vi "Create FTP Connection.vi"(8 "error in (no error)":errorcluster caption="错误输入（无错误）") -> (0 "error out":errorcluster caption="错误输出", 3 "TCP网络连接输出":T1)   [LabVIEW 2013]
uses:
  <vilib>/FTP/ftp0.llb/FTP Session.ctl
  <vilib>/FTP/NI_FTP.lvlib
panel:
  in  "port (21)":u16=21 caption="端口(21)"
  in  "password":string="success" caption="密码"
  in  "user":string="SUN Shouwang" caption="用户"
  in  "host IP":string="169.254.195.45" caption="主机IP"
  # "登陆信息"
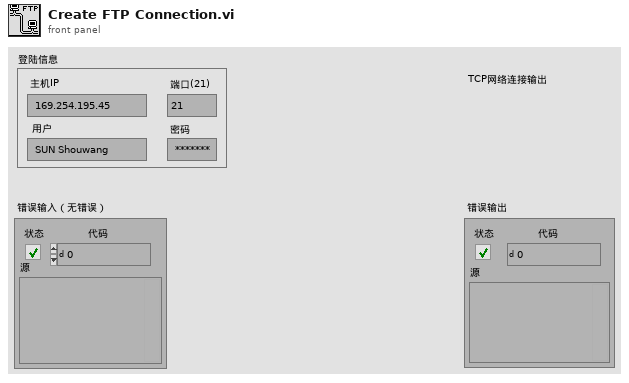
[diagram p1: front panel]
types:
  T1 = typedef "NI_FTP.lvlib/FTP Session.ctl" = refnum<k5>
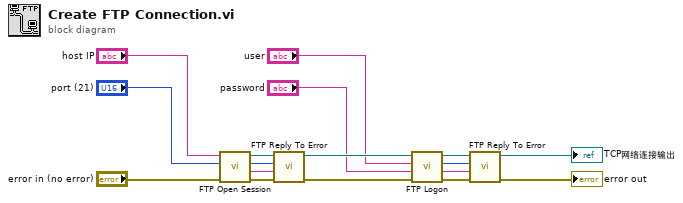
[diagram p0: block diagram]
diagram:
  n1 = call <vilib>:"FTP Open Session.vi"("error in (no error)"="error in (no error)", "remote port (21)"="port (21)", "address"="host IP") -> ("error out"=w7:errorcluster, "reply string"=w10:string, "reply code"=w9:i32, "ftp session"=w8:T1)  [unwired: 1 in, 4 out]
  n2 = call <vilib>:"FTP Reply To Error.vi"("error in (no error)"=w7, "reply string in"=w10, "reply code in"=w9, "ftp session"=w8) -> ("error out"=w12:errorcluster, "ftp session out"=w11:T1)  [unwired: 2 out]
  n3 = call <vilib>:"FTP Logon.vi"("error in (no error)"=w12, "password"="password", "user"="user", "ftp session"=w11) -> ("error out"=w13:errorcluster, "reply string"=w16:string, "reply code"=w15:i32, "ftp session out"=w14:T1)  [unwired: 4 out]
  n4 = call <vilib>:"FTP Reply To Error.vi"("error in (no error)"=w13, "reply string in"=w16, "reply code in"=w15, "ftp session"=w14) -> ("error out"=→"error out":errorcluster, "ftp session out"=→"TCP网络连接输出":T1)  [unwired: 2 out]
